vi "GetText.vi"(8 "error in":errorcluster, 11 "node in":refnum<class "PLTarget CVS.lvclass">) -> (0 "error out":errorcluster, 1 "additional text":string, 2 "text":string, 3 "node out":refnum<class "PLTarget CVS.lvclass">, 4 "glyph":string)   [LabVIEW 2013, in "PLTarget CVS.lvclass"]
doc: "Returns the text representation of the node used for the tree control."
uses:
  PLTarget CVS.lvclass
  Configuration Editor/Classes/Targets/Targets.lvclass
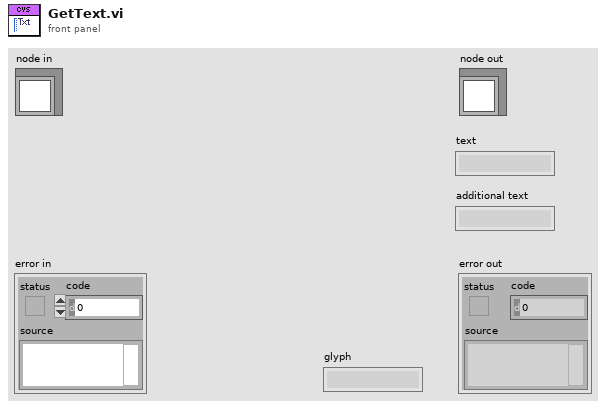
[diagram p1: front panel]
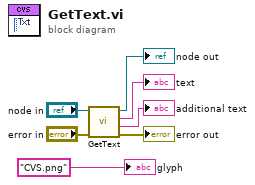
[diagram p0: block diagram]
diagram:
  n1 = call-parent "GetText.vi"("error in"="error in", "node in"="node in") -> ("error out"=→"error out":errorcluster, "additional text"=→"additional text":string, "text"=→"text":string, "node out"=→"node out":refnum<class "PLTarget CVS.lvclass">)  [unwired: 5 in, 1 out]
  "glyph" <- "CVS.png" ("Name")
